vi "AlliGator Sort Cursors for Square Gated IRF Fit.vi"(9 "Cursor Name Array in":string[](array[string]), 11 "Cursor Position Array in":dbl[](array[numeric])) -> (1 "Sorted Cursor Name Array":string[](array[string]), 3 "Sorted Cursor Position Array":dbl[](array[numeric]))   [LabVIEW 2021, in "AlliGator IRF.lvlib"]
doc: "Sorts 5 cursors by name (if they exist) corresponding to the 5 boundaries between regions in a square gate."
uses:
  AlliGator IRF.lvlib
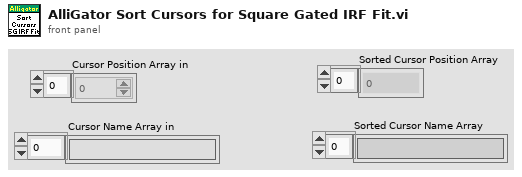
[diagram p1: front panel]
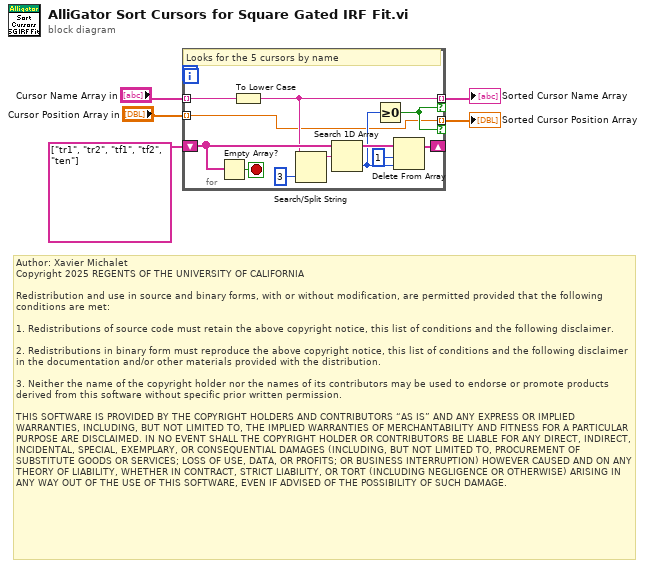
[diagram p0: block diagram]
diagram:
  # "Author: Xavier Michalet\nCopyright 2025 REGENTS OF THE UNIVERSITY OF CALIFORNIA\n\nRedistribution and use in source and binary forms, with or without modification, are permitted provided that the following conditions are met:\n\n1. Redistributions of source code must retain the above copyright notice, this list of conditions and the following disclaimer.\n\n2. Redistributions in binary form must reproduce the above copyright notice, this list of conditions and the following disclaimer in the documentation and/or other materials provided with the distribution.\n\n3. Neither the name of the copyright holder nor the names of its contributors may be used to endorse or promote products derived from this software without specific prior written permission.\n\nTHIS SOFTWARE IS PROVIDED BY THE COPYRIGHT HOLDERS AND CONTRIBUTORS “AS IS” AND ANY EXPRESS OR IMPLIED WARRANTIES, INCLUDING, BUT NOT LIMITED TO, THE IMPLIED WARRANTIES OF MERCHANTABILITY AND FITNESS FOR A PARTICULAR PURPOSE ARE DISCLAIMED. IN NO EVENT SHALL THE COPYRIGHT HOLDER OR CONTRIBUTORS BE LIABLE FOR ANY DIRECT, INDIRECT, INCIDENTAL, SPECIAL, EXEMPLARY, OR CONSEQUENTIAL DAMAGES (INCLUDING, BUT NOT LIMITED TO, PROCUREMENT OF SUBSTITUTE GOODS OR SERVICES; LOSS OF USE, DATA, OR PROFITS; OR BUSINESS INTERRUPTION) HOWEVER CAUSED AND ON ANY THEORY OF LIABILITY, WHETHER IN CONTRACT, STRICT LIABILITY, OR TORT (INCLUDING NEGLIGENCE OR OTHERWISE) ARISING IN ANY WAY OUT OF THE USE OF THIS SOFTWARE, EVEN IF ADVISED OF THE POSSIBILITY OF SUCH DAMAGE."
  n1 = for {
    tunnel: [w6] -> w4 mode=indexing if=w11
    shift-right: [w16] -> _
    shift-left: string[] ["tr1", "tr2", "tf1", "tf2", "ten"] -> [w14]
    tunnel: [w10] -> w3 mode=indexing if=w11
    tunnel: "Cursor Name Array in" -> [w7] mode=indexing
    tunnel: "Cursor Position Array in" -> [w6] mode=indexing
    stop <- w13 stop-if-true
    # "Looks for the 5 cursors by name"
    n2 = Empty Array?(array=w14) -> (empty?=w13:bool)
    n3 = To Lower Case(string=w7) -> (all lower case string=w10:string)
    n4 = Search/Split String(string=w10, offset (0)=3) -> (substring before match=w8:string)  [unwired: 1 in, 2 out]
    n5 = Search 1D Array(1D array=w14, element=w8) -> (index of element=w12:i32)  [unwired: 1 in]
    n6 = Greater Or Equal To 0?(x=w12) -> (x >= 0?=w11:bool)
    n7 = Delete From Array(array=w14, length=1, index=w12) -> (array with subset deleted=w16:string[])  [unwired: 1 out]
  }
  "Sorted Cursor Position Array" <- w4
  "Sorted Cursor Name Array" <- w3
